vi "Get Pin.vi"(0 "Serial Device in":refnum<class "Serial Device.lvclass">, 5 "VISA resource name":refnum<visa-resource-name>, 9 "Pin":u8, 11 "error in (no error)":errorcluster) -> (4 "Serial Device out":refnum<class "Serial Device.lvclass">, 6 "VISA resource name 2":refnum<visa-resource-name>, 8 "Boolean":bool, 10 "Response":string, 15 "error out":errorcluster)   [LabVIEW 2020, in "Serial Device.lvclass"]
doc: "GET PIN VI.\nEn este VI obtenemos el estado de el pin que el usuario desee dentro del microcontrolador elegido. Solo es posible obtener 4 pines de un puerto designado por el fabricante, que con facilidad puede ser modificado por el usuario"
uses:
  Serial Device.lvclass
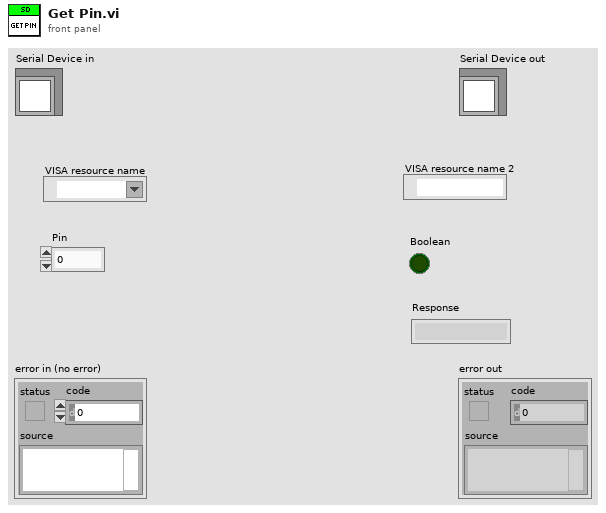
[diagram p1: front panel]
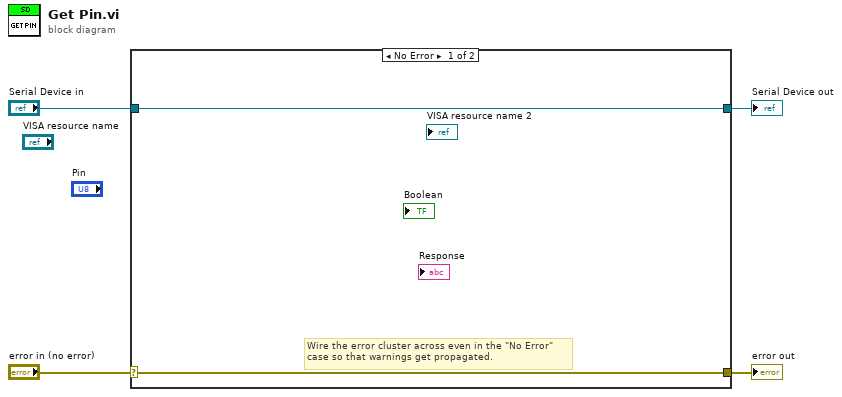
[diagram p0: block diagram]
diagram:
  n1 = case shown="No Error" "error in (no error)" {
    selector: "error in (no error)" -> [w5 w8]
    tunnel: [w5 w8] -> w3
    tunnel: [w6 w7] -> w1
    tunnel: "Serial Device in" -> [w6 w7]
    frame No Error {
      # "Wire the error cluster across even in the \"No Error\"\ncase so that warnings get propagated."
    }
    frame Error {
    }
  }
  "error out" <- w3
  "Serial Device out" <- w1
